vi "CRYPEAQ Corr.vi"(9 "M":dbl, 10 "NL":dbl, 11 "D":dbl[](array[numeric])) -> (3 "C":dbl[](array[numeric]))   [LabVIEW 2013]
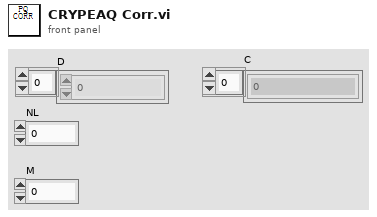
[diagram p1: front panel]
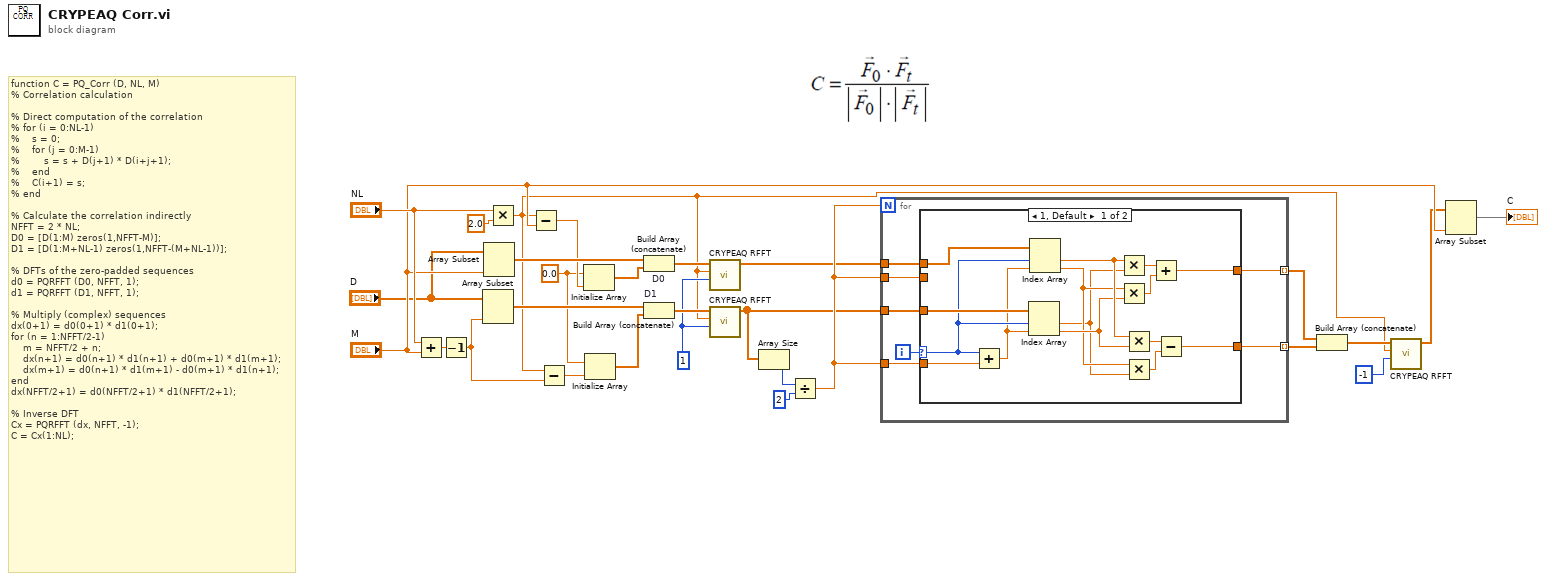
[diagram p0: block diagram]
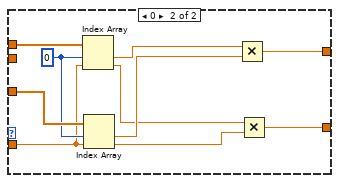
[diagram p2: hidden frame]
diagram:
  w9 = 1 ("ifn")
  w24 = 0.0 ("element")
  # "function C = PQ_Corr (D, NL, M)\n% Correlation calculation\n\n% Direct computation of the correlation\n% for (i = 0:NL-1)\n%    s = 0;\n%    for (j = 0:M-1)\n%        s = s + D(j+1) * D(i+j+1);\n%    end\n%    C(i+1) = s;\n% end\n\n% Calculate the correlation indirectly\nNFFT = 2 * NL;\nD0 = [D(1:M) zeros(1,NFFT-M)];\nD1 = [D(1:M+NL-1) zeros(1,NFFT-(M+NL-1))];\n\n% DFTs of the zero-padded sequences\nd0 = PQRFFT (D0, NFFT, 1);\nd1 = PQRFFT (D1, NFFT, 1);\n\n% Multiply (complex) sequences\ndx(0+1) = d0(0+1) * d1(0+1);\nfor (n = 1:NFFT/2-1)\n    m = NFFT/2 + n;\n    dx(n+1) = d0(n+1) * d1(n+1) + d0(m+1) * d1(m+1);\n    dx(m+1) = d0(n+1) * d1(m+1) - d0(m+1) * d1(n+1);\nend\ndx(NFFT/2+1) = d0(NFFT/2+1) * d1(NFFT/2+1);\n\n% Inverse DFT\nCx = PQRFFT (dx, NFFT, -1);\nC = Cx(1:NL);"
  n1 = Add(x="NL", y="M") -> (x+y=w13:dbl)
  n2 = Decrement(x=w13) -> (x-1=w12:dbl)
  n3 = Array Subset(array="D", length=w12) -> (w26:dbl[])  [unwired: 1 in]
  n4 = Array Subset(array="D", length="M") -> (w27:dbl[])  [unwired: 1 in]
  n5 = Multiply(x="NL", y=2.0) -> (x*y=w3:dbl)
  n6 = Subtract(x=w3, y="M") -> (x-y=w25:dbl)
  n7 = Subtract(x=w3, y=w12) -> (x-y=w23:dbl)
  n8 = Initialize Array(w24, w25) -> (w21:dbl[])
  n9 = Initialize Array(w24, w23) -> (w22:dbl[])
  n10 = Build Array (concatenate) "D0"(w27, w21) -> (w11:dbl[])
  n11 = Build Array (concatenate) "D1"(w26, w22) -> (w10:dbl[])
  n12 = call "CRYPEAQ RFFT.vi"("ifn"=w9, "N"=w3, "x"=w11) -> ("X"=w8:dbl[])  [unwired: 8 in]
  n13 = call "CRYPEAQ RFFT.vi"("ifn"=w9, "N"=w3, "x"=w10) -> ("X"=w7:dbl[])  [unwired: 8 in]
  n14 = Array Size(array=w7) -> (size(s)=w19:i32)
  n15 = Divide(x=w19, y=2) -> (x/y=w18:dbl)
  n16 = for {
    N: w18 -> [_]
    tunnel: w18 -> [w32]
    tunnel: [w31] -> w17 mode=indexing
    tunnel: w7 -> [w33]
    tunnel: w8 -> [w34]
    tunnel: w18 -> [w30]
    tunnel: [w29] -> w16 mode=indexing
    i -> [w35]
    n17 = case shown="1, Default" w35 {
      selector: w35 -> [w47 _]
      tunnel: w34 -> [w50 w60]
      tunnel: w33 -> [w49 w59]
      tunnel: w32 -> [_ _]
      tunnel: [w37 w56] -> w31
      tunnel: w30 -> [w46 w54]
      tunnel: [w36 w51] -> w29
      frame 1, Default {
        n18 = Add(x=w47, y=w46) -> (x+y=w45:dbl)
        n19 = Index Array(array=w49, index #1=w47, index #2=w45) -> (element #1=w38:dbl, element #2=w40:dbl)
        n20 = Index Array(array=w50, index #1=w47, index #2=w45) -> (element #1=w41:dbl, element #2=w39:dbl)
        n21 = Multiply(x=w41, y=w38) -> (x*y=w48:dbl)
        n22 = Multiply(x=w39, y=w40) -> (x*y=w44:dbl)
        n23 = Multiply(x=w41, y=w40) -> (x*y=w42:dbl)
        n24 = Multiply(x=w39, y=w38) -> (x*y=w43:dbl)
        n25 = Add(x=w48, y=w44) -> (x+y=w37:dbl)
        n26 = Subtract(x=w42, y=w43) -> (x-y=w36:dbl)
      }
      frame 0 {
        w55 = 0 ("index")
        n27 = Index Array(array=w60, index #1=w55, index #2=w54) -> (element #1=w58:dbl, element #2=w53:dbl)
        n28 = Index Array(array=w59, index #1=w55, index #2=w54) -> (element #1=w57:dbl, element #2=w52:dbl)
        n29 = Multiply(x=w58, y=w57) -> (x*y=w56:dbl)
        n30 = Multiply(x=w53, y=w52) -> (x*y=w51:dbl)
      }
    }
  }
  n31 = Build Array (concatenate)(w17, w16) -> (w5:dbl[])
  n32 = call "CRYPEAQ RFFT.vi"("ifn"=-1, "N"=w3, "x"=w5) -> ("X"=w2:dbl[])  [unwired: 8 in]
  n33 = Array Subset(array=w2, length="M") -> (→"C":dbl[])  [unwired: 1 in]
